vi "get_current_positions.vi"(0 "device_index (in) [0=def]":i32, 2 "axis":T1, 5 "Error In":errorcluster) -> (19 "Error Out":errorcluster)   [LabVIEW 2013, in "examples.lvlib"]
doc: "Demonstrates retrieving the pulse position at a specified index (for multi-axis) applications. In the case of single-axis applications, the axis input need not be wired.\n\nProduced By:\n\n<B>Kod Integrations, LLC</B>\n4835 Marianne Drive\nMount Airy, MD 21771\nhttp://www.kodintegrations.com\nemail: info@kodintegrations.com\nphone: (240) 687-1288"
uses:
  libraries/examples.lvlib
  classes/Controller/_Controller.lvclass
  common/controls/axis.ctl
  libraries/common.lvlib
panel:
  out "current_position (units)":i32
  in  "clear_buffer? (T)":bool=TRUE
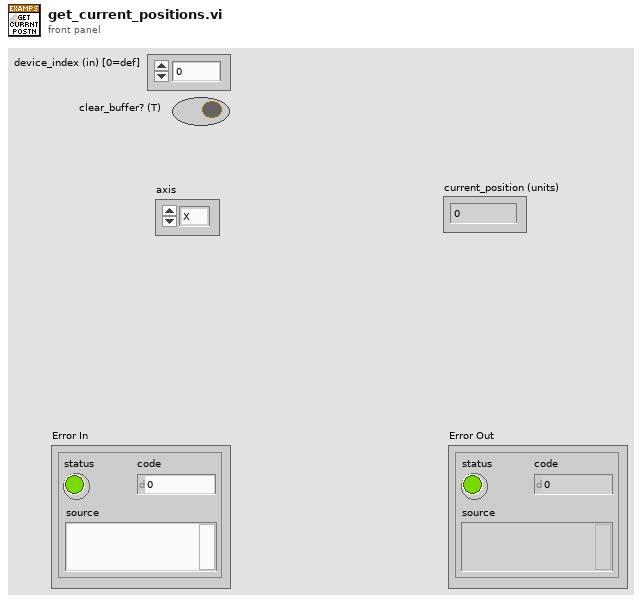
[diagram p1: front panel]
types:
  T1 = typedef "common.lvlib/axis.ctl" = enum16{"X", "Y", "Z", "U"}
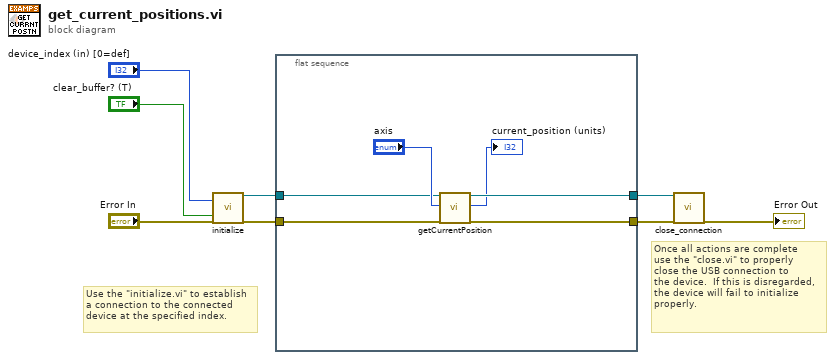
[diagram p0: block diagram]
diagram:
  # "Once all actions are complete\nuse the \"close.vi\" to properly\nclose the USB connection to \nthe device.  If this is disregarded,\nthe device will fail to initialize \nproperly."
  # "Use the \"initialize.vi\" to establish\na connection to the connected\ndevice at the specified index."
  n1 = call "initialize.vi"("device_index (in) [0=def]"="device_index (in) [0=def]", "clear_buffer? (T)"="clear_buffer? (T)", "error in (no error)"="Error In") -> ("reference (out)"=w5:refnum<class "_Controller.lvclass">, "error out"=w4:errorcluster)  [unwired: 15 in]
  n2 = flat-sequence {
    tunnel: w5 -> [w13]
    tunnel: w4 -> [w12]
    tunnel: [w11] -> w2
    tunnel: [w10] -> w1
    frame #0 {
      n3 = call-dynamic "getCurrentPosition.vi"("reference (in)"=w13, "axis (def=X)"="axis", "error in (no error)"=w12) -> ("reference (out)"=w11:refnum<class "_Controller.lvclass">, "current_position (units)"=→"current_position (units)":i32, "error out"=w10:errorcluster)  [unwired: 14 in]
    }
  }
  n4 = call "close_connection.vi"("reference (in)"=w2, "error in (no error)"=w1) -> ("error out"=→"Error Out":errorcluster)  [unwired: 16 in, 1 out]
